vi "main_target.vi"() -> ()   [LabVIEW 2011]
uses:
  controls.llb/command.ctl
  controls.llb/RTFIFO operate.ctl
panel:
  in  "variable":T2 {"command" items=["NO_Action", "start", "pause", "resum", "stop", "config"]}
  in  "error in":errorcluster
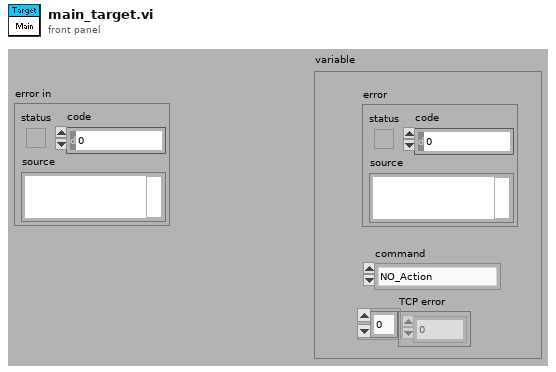
[diagram p1: front panel]
types:
  T1 = typedef "command.ctl" = u16
  T2 = cluster{"error":errorcluster, "TCP error":i32[], "command":T1}
  T3 = enum16{"connect", "receive data", "send data", "data transfer"}
  T4 = enum16{"connect", "receive data", "send data", "data transfer", "close"}
  T5 = typedef "RTFIFO operate.ctl" = enum16{"Creat", "Write", "Read", "Delete"}
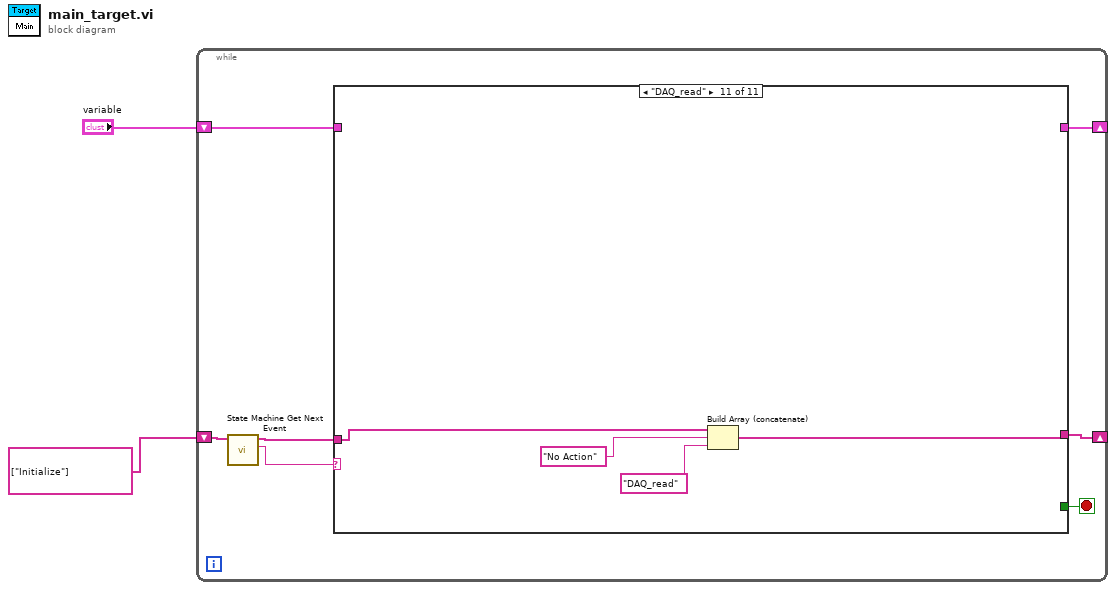
[diagram p0: block diagram]
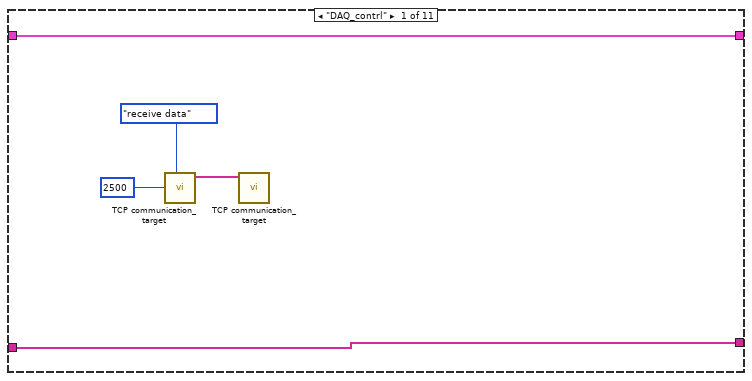
[diagram p2: hidden frame]
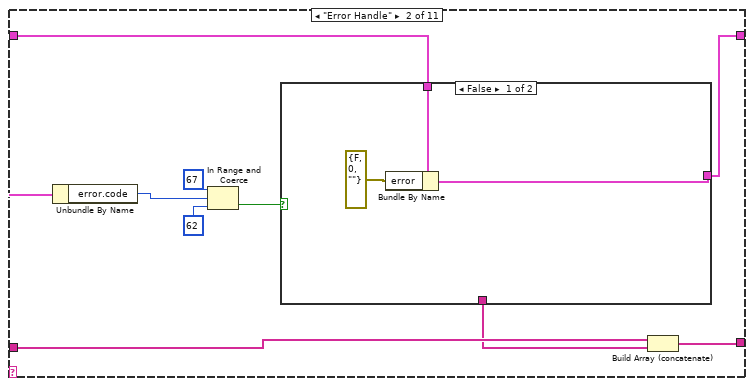
[diagram p3: hidden frame]
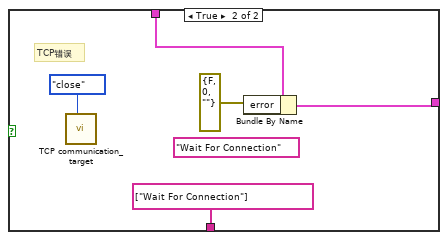
[diagram p4: hidden frame]
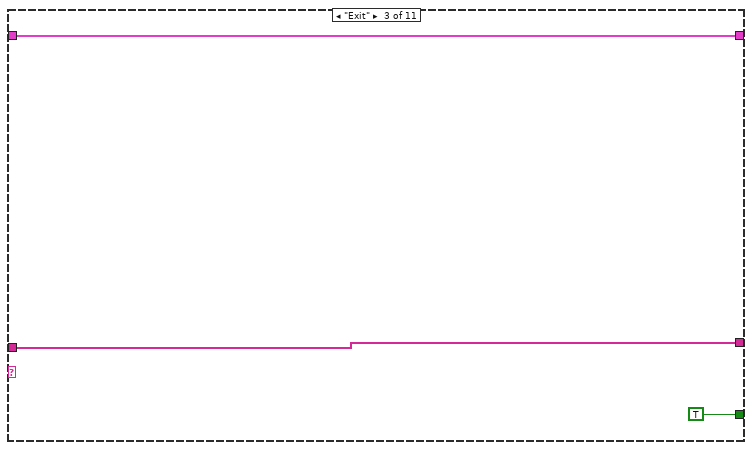
[diagram p5: hidden frame]
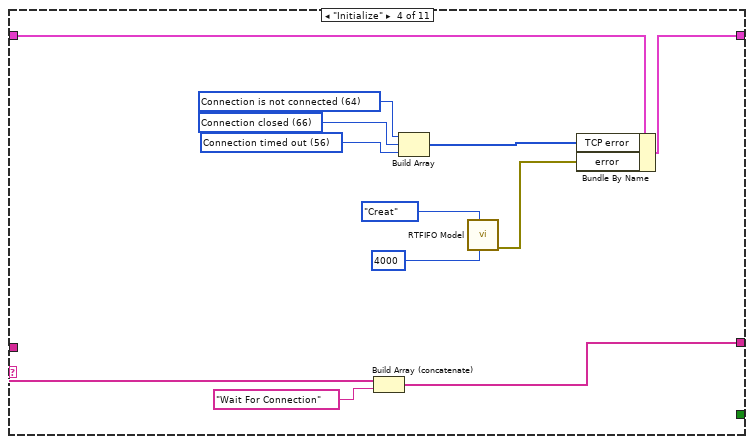
[diagram p6: hidden frame]
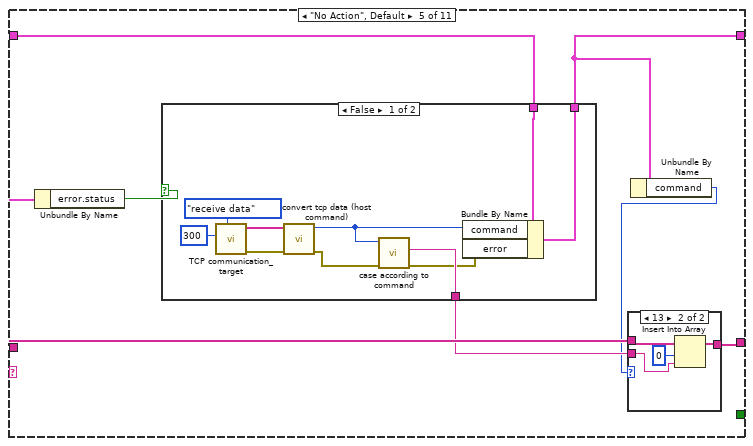
[diagram p7: hidden frame]
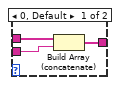
[diagram p8: hidden frame]
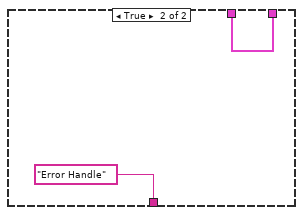
[diagram p9: hidden frame]
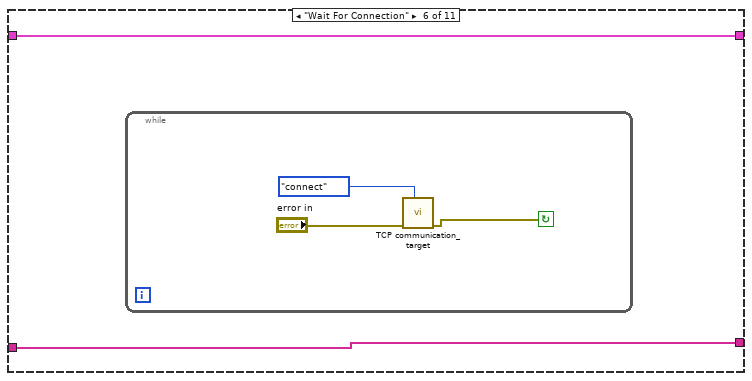
[diagram p10: hidden frame]
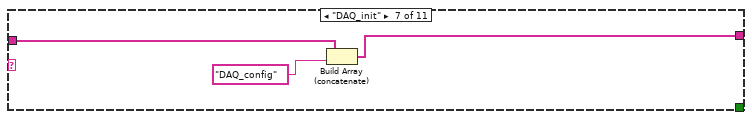
[diagram p11: hidden frame]
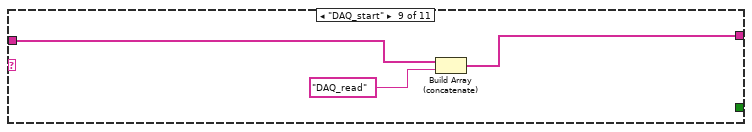
[diagram p13: hidden frame]
diagram:
  n1 = while {
    shift-right: [w5] -> _
    shift-left: string[] ["Initialize"] -> [w9]
    shift-right: [w3] -> _
    shift-left: "variable" -> [w4]
    stop <- w7 stop-if-true
    n2 = call "State Machine Get Next Event.vi"("event queue in"=w9) -> ("next event"=w8:string, "event queue out"=w6:string[])  [unwired: 5 in]
    n3 = case shown="\"DAQ_read\"" w8 {
      tunnel: [_ _ TRUE _ _ _ _ _ _ _ _] -> w7
      tunnel: w6 -> [w10 w21 w33 w46 w53 w74 w80 w81 w84 w86 w90]
      tunnel: [w10 w20 w33 w45 w52 w74 w79 w81 w82 w86 w89] -> w5
      tunnel: w4 -> [w14 w23 w32 w41 w51 w73 _ _ _ w85 _]
      tunnel: [w14 w22 w32 w40 w48 w73 _ _ _ w85 _] -> w3
      frame "DAQ_contrl" {
        n4 = call "TCP communication_target.vi"("TCP command"=T3."receive data", "timeout ms"=2500) -> ("Data out"=w11:string[])  [unwired: 8 in, 1 out]
        n5 = call "TCP communication_target.vi"("Data in"=w11) -> ()  [unwired: 9 in, 2 out]
      }
      frame "Error Handle" {
        n6 = Unbundle By Name(w23) -> ("error.code"=w18:i32)
        n7 = In Range and Coerce(upper limit=67, x=w18, lower limit=62) -> (In Range?=w15:bool)  [unwired: 1 out]
        n8 = case shown="False" w15 {
          tunnel: w23 -> [w26 w30]
          tunnel: [w24 w29] -> w22
          tunnel: [_ string[] ["Wait For Connection"]] -> w19
          frame False {
            n9 = Bundle By Name(cluster=w26, "error"=errorcluster {"status"=FALSE, "code"=0, "source"=""}) -> (w24:T2)
          }
          frame True {
            (unwired) "Wait For Connection"
            # "TCP错误"
            n10 = call "TCP communication_target.vi"("TCP command"=T4."close") -> ()  [unwired: 9 in, 2 out]
            n11 = Bundle By Name(cluster=w30, "error"=errorcluster {"status"=FALSE, "code"=0, "source"=""}) -> (w29:T2)
          }
        }
        n12 = Build Array (concatenate)(w21, w19) -> (w20:string[])
      }
      frame "Exit" {
      }
      frame "Initialize" {
        w38 = 66 items=["No Error", "Argument Error", "Memory Full", "Out of Zone", "End of File", "File Already Open", "Generic File IO Error", "File Not Found", "File Permission Error", "Disk Full", "Duplicate Path", "Too Many Files Open", "Not Enabled", "Resource File Not Found", "Cannot Add Resource", "Resource Not Found", "Image Not Found", "Image Memory Error", "Pen Does Not Exist", "Config Bad Type", "Config Token Not Found", "Config Parse Error", "Config Memory Error", "Bad External Code Format", "Bad External Code Offset", "External Code Not Present", "Null Window", "Destroy Window Mixup", "Null Menu", "Print Aborted", "Bad Print Record", "Print Driver Error", "Windows Error During Print", "Memory Error During Print", "Print Dialog Error", "Generic Print Error", "Invalid Device Refnum", "Device Not Found", "Device Parameter Error", "Device Unit Error", "Can't Open Device", "Device Call Aborted", "Generic Error", "Cancelled By User", "Object ID Too Low", "Object ID Too High", "Object Not In Heap", "Unknown Heap", "Bad DefProc ID", "DefProc Not In Table", "Message Out Of Range", "Null Method", "Unknown Message", "Manager Call Not Supported", "Bad address", "Connection In progress", "Connection timed out", "Connection is already in progress", "Network attribute not supported", "Network error", "Address in use", "System out of memory", "Connection aborted", "Connection refused", "Connection is not connected", "Connection is already connected", "Connection closed", "Initialize error (interapplication manager)", "Bad occurrence", "Wait on unbound occurrence handler", "Occurrence queue overflow", "Bad path", "Semaphore not signaled", "Unrecognized type (interapplication manager)"] ("1st Error to Convert")
        w37 = 56 items=["No Error", "Argument Error", "Memory Full", "Out of Zone", "End of File", "File Already Open", "Generic File IO Error", "File Not Found", "File Permission Error", "Disk Full", "Duplicate Path", "Too Many Files Open", "Not Enabled", "Resource File Not Found", "Cannot Add Resource", "Resource Not Found", "Image Not Found", "Image Memory Error", "Pen Does Not Exist", "Config Bad Type", "Config Token Not Found", "Config Parse Error", "Config Memory Error", "Bad External Code Format", "Bad External Code Offset", "External Code Not Present", "Null Window", "Destroy Window Mixup", "Null Menu", "Print Aborted", "Bad Print Record", "Print Driver Error", "Windows Error During Print", "Memory Error During Print", "Print Dialog Error", "Generic Print Error", "Invalid Device Refnum", "Device Not Found", "Device Parameter Error", "Device Unit Error", "Can't Open Device", "Device Call Aborted", "Generic Error", "Cancelled By User", "Object ID Too Low", "Object ID Too High", "Object Not In Heap", "Unknown Heap", "Bad DefProc ID", "DefProc Not In Table", "Message Out Of Range", "Null Method", "Unknown Message", "Manager Call Not Supported", "Bad address", "Connection In progress", "Connection timed out", "Connection is already in progress", "Network attribute not supported", "Network error", "Address in use", "System out of memory", "Connection aborted", "Connection refused", "Connection is not connected", "Connection is already connected", "Connection closed", "Initialize error (interapplication manager)", "Bad occurrence", "Wait on unbound occurrence handler", "Occurrence queue overflow", "Bad path", "Semaphore not signaled", "Unrecognized type (interapplication manager)"] ("1st Error to Convert")
        w39 = 64 items=["No Error", "Argument Error", "Memory Full", "Out of Zone", "End of File", "File Already Open", "Generic File IO Error", "File Not Found", "File Permission Error", "Disk Full", "Duplicate Path", "Too Many Files Open", "Not Enabled", "Resource File Not Found", "Cannot Add Resource", "Resource Not Found", "Image Not Found", "Image Memory Error", "Pen Does Not Exist", "Config Bad Type", "Config Token Not Found", "Config Parse Error", "Config Memory Error", "Bad External Code Format", "Bad External Code Offset", "External Code Not Present", "Null Window", "Destroy Window Mixup", "Null Menu", "Print Aborted", "Bad Print Record", "Print Driver Error", "Windows Error During Print", "Memory Error During Print", "Print Dialog Error", "Generic Print Error", "Invalid Device Refnum", "Device Not Found", "Device Parameter Error", "Device Unit Error", "Can't Open Device", "Device Call Aborted", "Generic Error", "Cancelled By User", "Object ID Too Low", "Object ID Too High", "Object Not In Heap", "Unknown Heap", "Bad DefProc ID", "DefProc Not In Table", "Message Out Of Range", "Null Method", "Unknown Message", "Manager Call Not Supported", "Bad address", "Connection In progress", "Connection timed out", "Connection is already in progress", "Network attribute not supported", "Network error", "Address in use", "System out of memory", "Connection aborted", "Connection refused", "Connection is not connected", "Connection is already connected", "Connection closed", "Initialize error (interapplication manager)", "Bad occurrence", "Wait on unbound occurrence handler", "Occurrence queue overflow", "Bad path", "Semaphore not signaled", "Unrecognized type (interapplication manager)"] ("1st Error to Convert")
        n13 = Build Array (concatenate)(w46, "Wait For Connection") -> (w45:string[])
        n14 = Build Array(w39, w38, w37) -> (w36:i32[])
        n15 = call "RTFIFO Model.vi"("size"=4000, "operate"=RTFIFO_operate."Creat") -> ("error out"=w35:errorcluster)  [unwired: 8 in, 1 out]
        n16 = Bundle By Name(cluster=w41, "TCP error"=w36, "error"=w35) -> (w40:T2)
      }
      frame "No Action", Default {
        n17 = Unbundle By Name(w51) -> ("error.status"=w50:bool)
        n18 = case shown="False" w50 {
          tunnel: [w66 w71] -> w48
          tunnel: w51 -> [w65 w71]
          tunnel: [w64 "Error Handle"] -> w49
          frame False {
            n19 = call "TCP communication_target.vi"("TCP command"=T3."receive data", "timeout ms"=300) -> ("error out"=w68:errorcluster, "Data out"=w69:string[])  [unwired: 8 in]
            n20 = call "convert tcp data (host command).vi"("error in"=w68, "TCP Data"=w69) -> ("error out"=w63:errorcluster, "command"=w61:T1)  [unwired: 8 in]
            n21 = call "case according to command.vi"("error in"=w63, "command"=w61) -> ("error out"=w62:errorcluster, "case"=w64:string)  [unwired: 8 in]
            n22 = Bundle By Name(cluster=w65, "command"=w61, "error"=w62) -> (w66:T2)
          }
          frame True {
          }
        }
        n23 = Unbundle By Name(w48) -> ("command"=w47:T1)
        n24 = case shown="13" w47 {
          tunnel: w53 -> [w56 w60]
          tunnel: [w55 w57] -> w52
          tunnel: w49 -> [w54 w59]
          frame 0, Default {
            n25 = Build Array (concatenate)(w56, w54) -> (w55:string[])
          }
          frame 13 {
            n26 = Insert Into Array(array=w60, index=0, new element=w59) -> (w57:string[])
          }
        }
      }
      frame "Wait For Connection" {
        n27 = while {
          stop <- w77 continue-if-true
          n28 = call "TCP communication_target.vi"("TCP command"=T3."connect", "error in"="error in") -> ("error out"=w77:errorcluster)  [unwired: 8 in, 1 out]
        }
      }
      frame "DAQ_init" {
        n29 = Build Array (concatenate)(w80, "DAQ_config") -> (w79:string[])
      }
      frame "DAQ_config" {
      }
      frame "DAQ_start" {
        n30 = Build Array (concatenate)(w84, "DAQ_read" ("string")) -> (w82:string[])
      }
      frame "DAQ_stop" {
      }
      frame "DAQ_read" {
        n31 = Build Array (concatenate)(w90, "No Action", "DAQ_read" ("element")) -> (w89:string[])
      }
    }
  }
